vi "Circle Area Perimeter.vi"() -> ()   [LabVIEW 2019]
panel:
  in  "r":dbl
  out "Area":dbl
  out "Perimeter":dbl
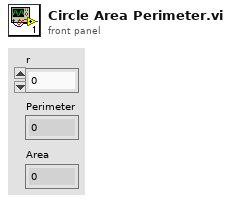
[diagram p1: front panel]
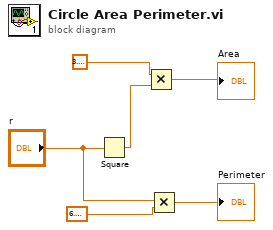
[diagram p0: block diagram]
diagram:
  n1 = Square(x="r") -> (x^2=w4:dbl)
  n2 = Multiply(x=3.141592653589793, y=w4) -> (x*y=→"Area":dbl)
  n3 = Multiply(x="r", y=6.283185307179586) -> (x*y=→"Perimeter":dbl)
